vi "Number of Retry Connection--constant.vi"() -> (0 "Number of Retry":i32=5)   [LabVIEW 2024, in "EtherCAT Model.lvlib"]
uses:
  EtherCAT Model.lvlib
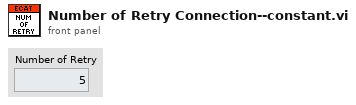
[diagram p1: front panel]
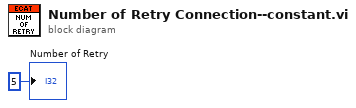
[diagram p0: block diagram]
diagram:
  "Number of Retry" <- 5
